vi "Configure Identity.vi"(8 "error in (no error)":errorcluster, 10 "Model Number (0: E3631XA)":i32(ring) items=["E3631XA", "E3631A"], 11 "VISA resource name":refnum<visa-resource-name>) -> (0 "error out":errorcluster, 3 "VISA resource name out":refnum<visa-resource-name>)   [LabVIEW 2020, in "Keysight E36300 Series.lvlib"]
doc: "Configures the model number.\n\n<b>Note:</b>\nThis VI will change the mainframe model ID string for backward compatibility.\nThis VI is not applicable for EDU36311A model."
uses:
  Keysight E36300 Series.lvlib
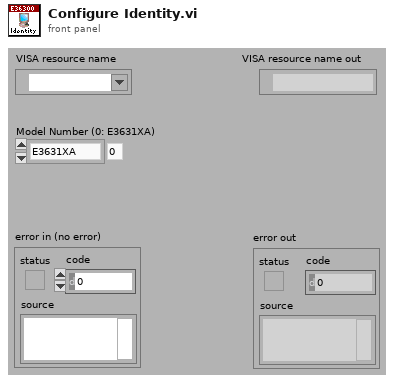
[diagram p1: front panel]
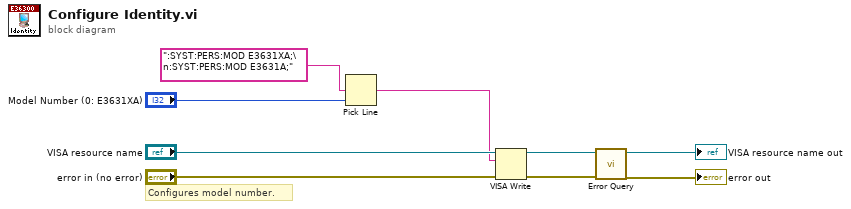
[diagram p0: block diagram]
diagram:
  # "Configures model number."
  n1 = Pick Line(multi-line string=":SYST:PERS:MOD E3631XA;\n:SYST:PERS:MOD E3631A;", line index="Model Number (0: E3631XA)") -> (output string=w1:string)  [unwired: 1 in]
  n2 = VISA Write(VISA resource name="VISA resource name", write buffer=w1, error in (no error)="error in (no error)") -> (VISA resource name out=w5:refnum<visa-resource-name>, error out=w4:errorcluster)  [unwired: 1 out]
  n3 = call "Error Query.vi"("error in (no error)"=w4, "VISA resource name"=w5) -> ("error out"=→"error out":errorcluster, "VISA resource name out"=→"VISA resource name out":refnum<visa-resource-name>)  [unwired: 6 in, 2 out]
